vi "checkCmdIdOrder.vi"(8 "error in (no error)":errorcluster, 10 "jsonCmd":string, 11 "tcpServer in":refnum<class "TcpServer.lvclass">) -> (0 "error out":errorcluster, 2 "ok":bool, 3 "tcpServer out":refnum<class "TcpServer.lvclass">)   [LabVIEW 2018, in "TcpServer.lvclass"]
doc: "Check the cmdId is bigger then the previous, if is not the first command."
uses:
  TcpServer.lvclass
panel:
  out "penultimate":i32
  out "latest":i32
  in  "Init array":i32[](array[numeric])
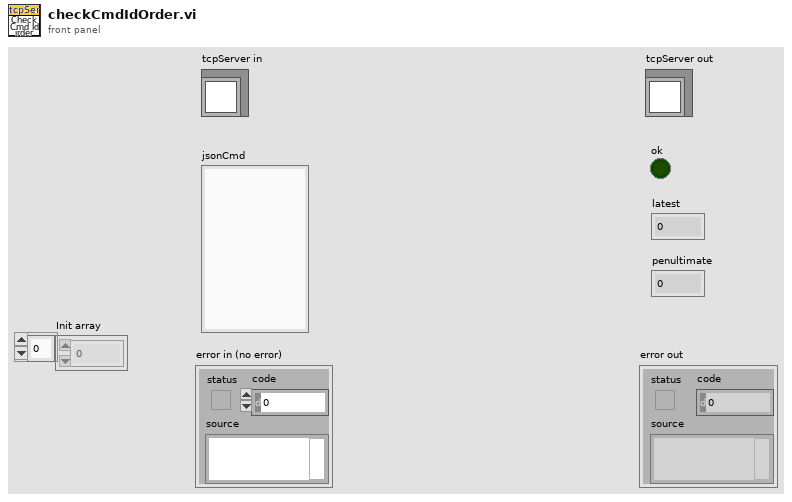
[diagram p1: front panel]
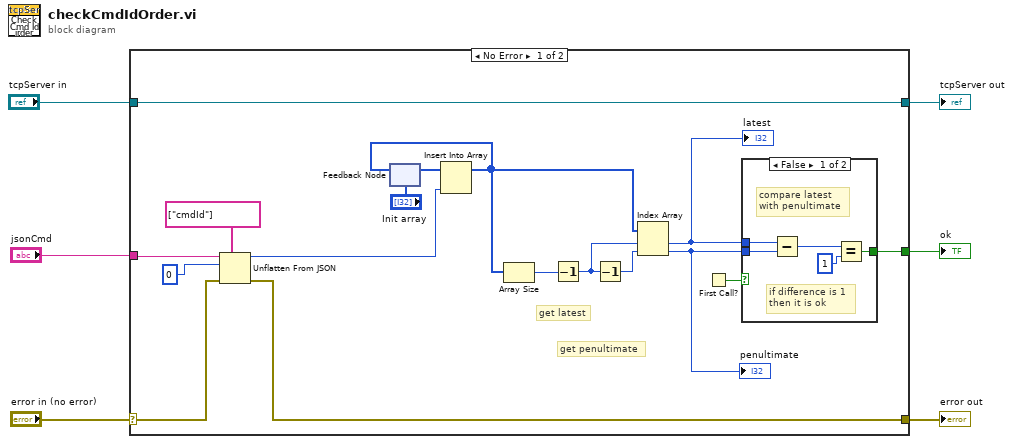
[diagram p0: block diagram]
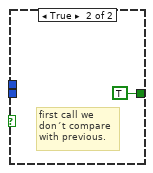
[diagram p2: hidden frame]
diagram:
  n1 = case shown="No Error" "error in (no error)" {
    selector: "error in (no error)" -> [w12 w31]
    tunnel: [w11 w31] -> w5
    tunnel: "jsonCmd" -> [w13 _]
    tunnel: "tcpServer in" -> [w10 w30]
    tunnel: [w10 w30] -> w2
    tunnel: [w9 _] -> w1
    frame No Error {
      # "get penultimate"
      # "get latest"
      n2 = Unflatten From JSON(path=string[] ["cmdId"], JSON string=w13, type and defaults=0, error in (no error)=w12) -> (value=w7:i32, error out=w11:errorcluster)  [unwired: 3 in]
      n3 = feedback #1("Init array") -> (w23:i32[])
      n4 = Insert Into Array(array=w23, new element=w7) -> (w21:i32[])  [unwired: 1 in]
      n5 = feedback-in #1(w21) -> ()
      n6 = Array Size(array=w21) -> (size(s)=w20:i32)
      n7 = Decrement(x=w20) -> (x-1=w19:i32)
      n8 = Decrement(x=w19) -> (x-1=w18:i32)
      n9 = Index Array(array=w21, index #1=w19, index #2=w18) -> (element #1=w17:i32, element #2=w16:i32)
      "latest" <- w17
      "penultimate" <- w16
      n10 = First Call?() -> (First Call?: T/F=w15:bool)
      n11 = case shown="False" w15 {
        tunnel: w17 -> [w28 _]
        tunnel: w16 -> [w27 _]
        tunnel: [w24 TRUE] -> w9
        frame False {
          # "compare latest\nwith penultimate"
          # "if difference is 1\nthen it is ok"
          n12 = Subtract(x=w28, y=w27) -> (x-y=w26:i32)
          n13 = Equal?(x=w26, y=1) -> (x = y?=w24:bool)
        }
        frame True {
          # "first call we\ndon´t compare\nwith previous."
        }
      }
    }
    frame Error {
    }
  }
  "error out" <- w5
  "tcpServer out" <- w2
  "ok" <- w1
